vi "Pre Launch Init.vi"(11 "Mixer in":refnum<class "Mixer.lvclass">) -> (0 "error out":errorcluster, 3 "Mixer out":refnum<class "Mixer.lvclass">)   [LabVIEW 2018, in "Feeder Actor.lvlib" / "Mixer.lvclass"]
doc: "(<B>Filename</B>: Actor Framework.lvlib:Actor.lvclass:Pre Launch Init.vi)\n\nDefines behavior that occurs after the Launch Nested Actor method is invoked but before the actor's Actor Core method begins running.\n\nBy default, this method does nothing. A descendant class may override it to define behavior."
uses:
  Mixer.lvclass
  Mixer.lvclass/Mixer.ctl
  <vilib>/DAQmx/create/channels.llb/DAQmx Create Channel (CO-Pulse Generation-Frequency).vi
  <vilib>/DAQmx/configure/timing.llb/DAQmx Timing (Implicit).vi
  <vilib>/MGI/Panel Manager/Panel Actor/Panel Actor/Panel Actor.lvclass
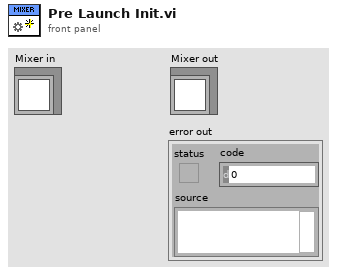
[diagram p1: front panel]
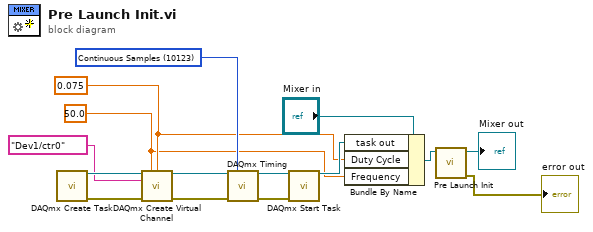
[diagram p0: block diagram]
diagram:
  w2 = 0.075 ("duty cycle")
  w1 = 50.0 ("frequency")
  w8 = 10123 items=["Finite Samples"=10178, "Continuous Samples"=10123, "Hardware Timed Single Point"=12522] ("sample mode")
  n1 = call <vilib>:"DAQmx Create Task.vi"() -> ("task out"=w11:refnum<k21>, "error out"=w12:errorcluster)  [unwired: 14 in]
  n2 = call-poly <vilib>:"DAQmx Create Virtual Channel.vi"("task in"=w11, "frequency"=w1, "duty cycle"=w2, "counter"=tag "Dev1/ctr0" ("Counter(s)"), "error in"=w12) -> ("task out"=w9:refnum<k21>, "error out"=w10:errorcluster)  [unwired: 9 in]
  n3 = call-poly <vilib>:"DAQmx Timing.vi"("task/channels in"=w9, "sample mode"=w8, "error in"=w10) -> ("task out"=w13:refnum<k21>, "error out"=w14:errorcluster)  [unwired: 11 in]
  n4 = call <vilib>:"DAQmx Start Task.vi"("task/channels in"=w13, "error in"=w14) -> ("task out"=w5:refnum<k21>)  [unwired: 12 in, 1 out]
  n5 = Bundle By Name(cluster="Mixer in", "task out"=w5, "Duty Cycle"=w2, "Frequency"=w1) -> (w4:refnum<class "Mixer.lvclass">)
  n6 = call-parent "Pre Launch Init.vi"("Panel Actor in"=w4) -> ("error out"=→"error out":errorcluster, "Panel Actor out"=→"Mixer out":refnum<class "Mixer.lvclass">)  [unwired: 9 in]
